vi "告警处理.vi"() -> ()   [LabVIEW 2016, in "main.lvlib"]
uses:
  main.lvlib
  <vilib>/ptbypt/NI_PtbyPt.lvlib
  bbe/bbe.lvlib
  EXO2/EXO2.lvlib
panel:
  out "millisecond timer value 4":u32
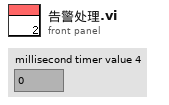
[diagram p1: front panel]
types:
  T1 = typedef "报警信息字段定义.ctl" = cluster{"时间":timestamp, "参数":string, "元器件":string, "故障现象":string, "故障分析":string, "state":string, "code":string, "platform_alarm_code":string}
  T2 = typedef "数据库类型.ctl" = enum16{"Access", "SQLite"}
  T3 = cluster{"Time":timestamp, "Temp":dbl, "SpCond":dbl, "Cond":dbl, "Sal":dbl, "TDS":dbl, "pH":dbl, "pH mV":dbl, "orp":dbl, "ODO %":dbl, "ODO mg/L":dbl, "Turb":dbl, "Chl":dbl, "Depth":dbl}
  T4 = cluster{"时间":timestamp, "Temp [℃]":dbl, "Green Algae [μg/L]":dbl, "Bluegreen [μg/L]":dbl, "Diatoms [μg/L]":dbl, "Cryptophyta [μg/L]":dbl, "Yellow substances [r.u.]":dbl, "Total Conc [μg/L]":dbl, "Transmission [%]":dbl, "Depth [m]":dbl}
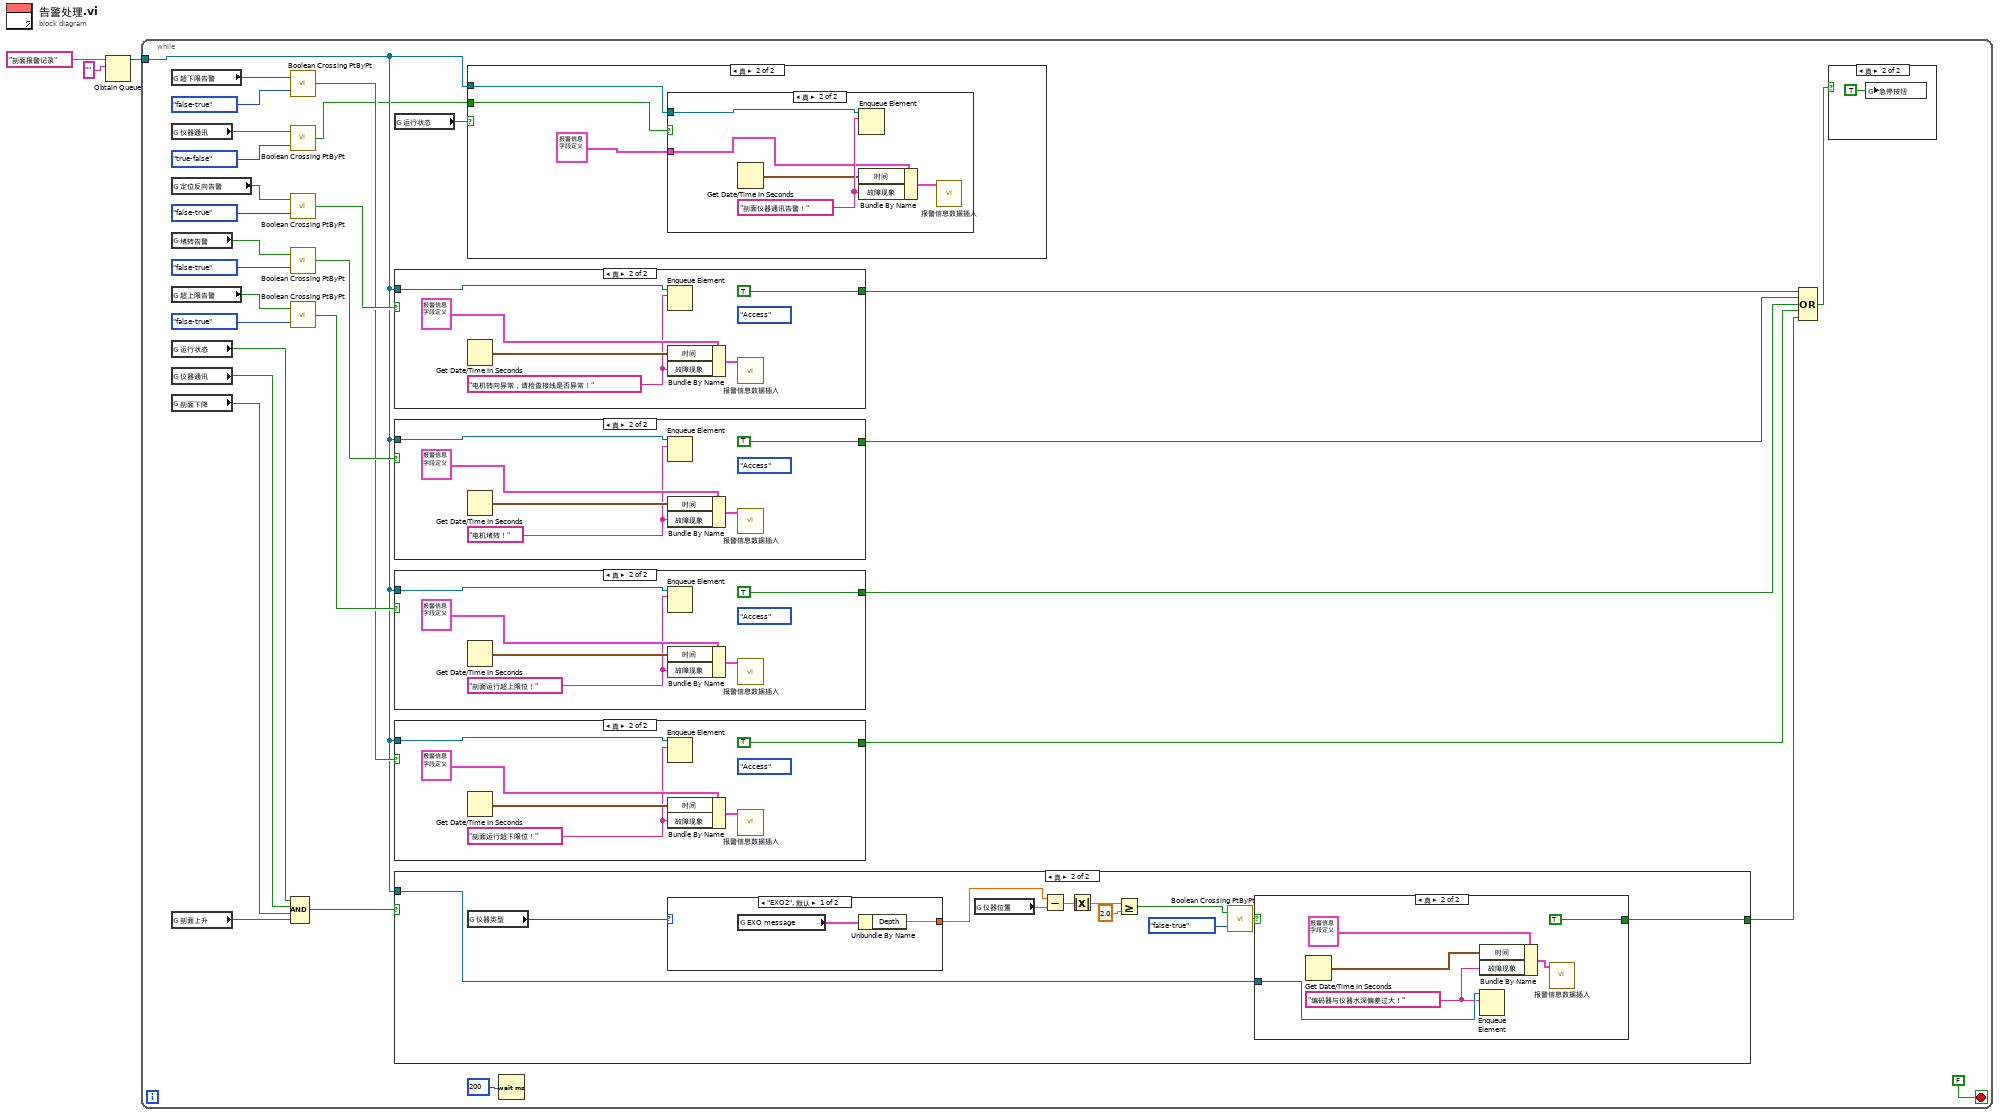
[diagram p0: block diagram]
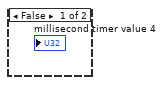
[diagram p4: hidden frame]
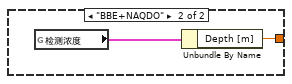
[diagram p6: hidden frame]
diagram:
  n1 = Obtain Queue(name (unnamed)="剖面报警记录" ("名称（未命名）"), element data type="") -> (queue out=w2:refnum<queue>)  [unwired: 3 in, 2 out]
  n2 = while {
    tunnel: w2 -> [w12]
    stop <- FALSE stop-if-true
    n3 = global read "全局非断电保持变量.vi" "超下限告警"() -> (w6:bool)
    n4 = global read "全局非断电保持变量.vi" "仪器通讯"() -> (w10:bool)
    n5 = global read "全局非断电保持变量.vi" "定位反向告警"() -> (w4:bool)
    n6 = global read "全局非断电保持变量.vi" "堵转告警"() -> (w5:bool)
    n7 = global read "全局非断电保持变量.vi" "超上限告警"() -> (w7:bool)
    n8 = global read "全局非断电保持变量.vi" "运行状态"() -> (w18:bool)
    n9 = global read "全局非断电保持变量.vi" "仪器通讯"() -> (w11:bool)
    n10 = global read "全局非断电保持变量.vi" "剖面下降"() -> (w15:bool)
    n11 = global read "全局非断电保持变量.vi" "剖面上升"() -> (w14:bool)
    n12 = call <vilib>:"Boolean Crossing PtByPt.vi"("direction"=enum16{"either", "false-true", "true-false"}."false-true", "input"=w6) -> ("crossing"=w21:bool)  [unwired: 1 in]
    n13 = call <vilib>:"Boolean Crossing PtByPt.vi"("direction"=enum16{"either", "false-true", "true-false"}."true-false", "input"=w10) -> ("crossing"=w8:bool)  [unwired: 1 in]
    n14 = call <vilib>:"Boolean Crossing PtByPt.vi"("direction"=enum16{"either", "false-true", "true-false"}."false-true", "input"=w4) -> ("crossing"=w30:bool)  [unwired: 1 in]
    n15 = call <vilib>:"Boolean Crossing PtByPt.vi"("direction"=enum16{"either", "false-true", "true-false"}."false-true", "input"=w5) -> ("crossing"=w29:bool)  [unwired: 1 in]
    n16 = call <vilib>:"Boolean Crossing PtByPt.vi"("direction"=enum16{"either", "false-true", "true-false"}."false-true", "input"=w7) -> ("crossing"=w23:bool)  [unwired: 1 in]
    n17 = Compound Arithmetic op=AND ("复合运算")(w18, w11, w15, w14) -> (w17:bool)
    n18 = global read "全局非断电保持变量.vi" "运行状态"() -> (w13:bool)
    n19 = case shown="真" w30 {
      tunnel: w12 -> [_ w87]
      tunnel: [_ TRUE] -> w27
      frame False {
      }
      frame True {
        (unwired) 数据库类型."Access" ("数据库类型")
        w82 = "电机转向异常，请检查接线是否异常！" ("元素")
        n20 = Get Date/Time In Seconds() -> (seconds since 1Jan1904=w85:timestamp)
        n21 = Enqueue Element(queue=w87, element=w82) -> ()  [unwired: 2 in, 3 out]
        n22 = Bundle By Name(cluster=T1 {"时间"=timestamp(0 s since 1904-01-01), "参数"="剖面系统", "元器件"="", "故障现象"="", "故障分析"="", "state"="", "code"="", "platform_alarm_code"=""} ("data"), "时间"=w85, "故障现象"=w82) -> (w84:T1)
        n23 = call "报警信息数据插入.vi"("data"=w84) -> ()  [unwired: 9 in, 1 out]
      }
    }
    n24 = case shown="真" w29 {
      tunnel: w12 -> [_ w81]
      tunnel: [_ TRUE] -> w26
      frame False {
      }
      frame True {
        (unwired) 数据库类型."Access" ("数据库类型")
        w76 = "电机堵转！" ("元素")
        n25 = Get Date/Time In Seconds() -> (seconds since 1Jan1904=w79:timestamp)
        n26 = Enqueue Element(queue=w81, element=w76) -> ()  [unwired: 2 in, 3 out]
        n27 = Bundle By Name(cluster=T1 {"时间"=timestamp(0 s since 1904-01-01), "参数"="剖面系统", "元器件"="", "故障现象"="", "故障分析"="", "state"="", "code"="", "platform_alarm_code"=""} ("data"), "时间"=w79, "故障现象"=w76) -> (w78:T1)
        n28 = call "报警信息数据插入.vi"("data"=w78) -> ()  [unwired: 9 in, 1 out]
      }
    }
    n29 = case shown="真" w23 {
      tunnel: w12 -> [_ w74]
      tunnel: [_ TRUE] -> w20
      frame False {
      }
      frame True {
        (unwired) 数据库类型."Access" ("数据库类型")
        w69 = "剖面运行超上限位！" ("元素")
        n30 = Get Date/Time In Seconds() -> (seconds since 1Jan1904=w72:timestamp)
        n31 = Enqueue Element(queue=w74, element=w69) -> ()  [unwired: 2 in, 3 out]
        n32 = Bundle By Name(cluster=T1 {"时间"=timestamp(0 s since 1904-01-01), "参数"="剖面系统", "元器件"="", "故障现象"="", "故障分析"="", "state"="", "code"="", "platform_alarm_code"=""} ("data"), "时间"=w72, "故障现象"=w69) -> (w71:T1)
        n33 = call "报警信息数据插入.vi"("data"=w71) -> ()  [unwired: 9 in, 1 out]
      }
    }
    n34 = case shown="真" w21 {
      tunnel: w12 -> [_ w68]
      tunnel: [_ TRUE] -> w19
      frame False {
      }
      frame True {
        (unwired) 数据库类型."Access" ("数据库类型")
        w63 = "剖面运行超下限位！" ("元素")
        n35 = Get Date/Time In Seconds() -> (seconds since 1Jan1904=w66:timestamp)
        n36 = Enqueue Element(queue=w68, element=w63) -> ()  [unwired: 2 in, 3 out]
        n37 = Bundle By Name(cluster=T1 {"时间"=timestamp(0 s since 1904-01-01), "参数"="剖面系统", "元器件"="", "故障现象"="", "故障分析"="", "state"="", "code"="", "platform_alarm_code"=""} ("data"), "时间"=w66, "故障现象"=w63) -> (w65:T1)
        n38 = call "报警信息数据插入.vi"("data"=w65) -> ()  [unwired: 9 in, 1 out]
      }
    }
    n39 = case shown="真" w17 {
      tunnel: w12 -> [_ w52]
      tunnel: [_ w51] -> w16
      frame False {
      }
      frame True {
        n40 = global read "全局断电保存变量.vi" "仪器类型"() -> (w50:enum16{"EXO2", "BBE+NAQDO"})
        n41 = case shown="\"EXO2\", 默认" w50 {
          tunnel: [w59 w61] -> w48
          frame "EXO2", Default {
            n42 = global read "EXO2全局变量.vi" "EXO message"() -> (w60:T3)
            n43 = Unbundle By Name(w60) -> ("Depth"=w59:dbl)
          }
          frame "BBE+NAQDO" {
            n44 = global read "过程变量.vi" "检测浓度"() -> (w62:T4)
            n45 = Unbundle By Name(w62) -> ("Depth [m]"=w61:dbl)
          }
        }
        n46 = global read "全局非断电保持变量.vi" "仪器位置"() -> (w49:dbl)
        n47 = Subtract(x=w48, y=w49) -> (x-y=w47:dbl)
        n48 = Absolute Value(x=w47) -> (abs(x)=w46:dbl)
        n49 = Greater Or Equal?(x=w46, y=2.0) -> (x >= y?=w43:bool)
        n50 = call <vilib>:"Boolean Crossing PtByPt.vi"("direction"=enum16{"either", "false-true", "true-false"}."false-true", "input"=w43) -> ("crossing"=w42:bool)  [unwired: 1 in]
        n51 = case shown="真" w42 {
          tunnel: w52 -> [_ w58]
          tunnel: [_ TRUE] -> w51
          frame False {
          }
          frame True {
            w53 = "编码器与仪器水深偏差过大！" ("元素")
            n52 = Get Date/Time In Seconds() -> (seconds since 1Jan1904=w56:timestamp)
            n53 = Bundle By Name(cluster=T1 {"时间"=timestamp(0 s since 1904-01-01), "参数"="剖面系统", "元器件"="", "故障现象"="", "故障分析"="", "state"="", "code"="", "platform_alarm_code"=""} ("data"), "时间"=w56, "故障现象"=w53) -> (w55:T1)
            n54 = Enqueue Element(queue=w58, element=w53) -> ()  [unwired: 2 in, 3 out]
            n55 = call "报警信息数据插入.vi"("data"=w55) -> ()  [unwired: 9 in, 1 out]
          }
        }
      }
    }
    n56 = case shown="真" w13 {
      tunnel: w12 -> [_ w36]
      tunnel: w8 -> [_ w35]
      frame False {
      }
      frame True {
        n57 = case shown="真" w35 {
          tunnel: w36 -> [_ w38]
          tunnel: T1 {"时间"=timestamp(0 s since 1904-01-01), "参数"="剖面系统", "元器件"="", "故障现象"="", "故障分析"="", "state"="", "code"="", "platform_alarm_code"=""} ("data") -> [_ w37]
          frame False {
          }
          frame True {
            w41 = "剖面仪器通讯告警！" ("元素")
            n58 = Get Date/Time In Seconds() -> (seconds since 1Jan1904=w39:timestamp)
            n59 = Enqueue Element(queue=w38, element=w41) -> ()  [unwired: 2 in, 3 out]
            n60 = Bundle By Name(cluster=w37, "时间"=w39, "故障现象"=w41) -> (w40:T1)
            n61 = call "报警信息数据插入.vi"("data"=w40) -> ()  [unwired: 9 in, 1 out]
          }
        }
      }
    }
    n62 = Wait (ms)(milliseconds to wait=u32 200 ("等待时间（毫秒）")) -> ()  [unwired: 1 out]
    n63 = Compound Arithmetic op=OR ("复合运算")(w27, w26, w20, w19, w16) -> (w25:bool)
    n64 = case shown="真" w25 {
      frame False {
      }
      frame True {
        n65 = global write "全局非断电保持变量.vi" "急停按钮"(TRUE ("急停按钮")) -> ()
      }
    }
  }
